vi "Test Pick and Place.vi"() -> ()   [LabVIEW 2011]
uses:
  Config Manager Class/Type Definitions/Fiducial Type.ctl
  Config Manager Class/Type Definitions/Part Type.ctl
  Gantry Class/Gantry Class.lvclass
  CameraTool Class/CameraTool Class.lvclass
  WorkTable Class/WorkTable Class.lvclass
  PickerTool Class.lvclass
  Config Manager Class/Config Manager Class.lvclass
panel:
  out "error out":errorcluster
  in  "BBM Slot":i32
  in  "HDI Slot":i32
  in  "BBM Chuck":i32=1
  in  "HDI Chuck":i32=4
  in  "Virtual Mode":bool
  in  "Config Folder":path=path "C:/Users/husker/Desktop/gantry/Config"
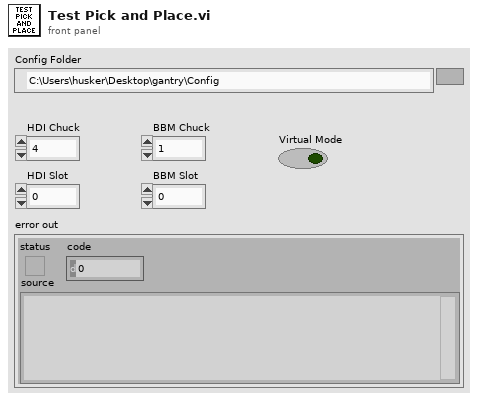
[diagram p1: front panel]
types:
  T1 = typedef "Fiducial Type.ctl" = enum16{"HDI", "BBM"}
  T2 = typedef "Part Type.ctl" = enum16{"BBM", "HDI", "BARE HDI", "GLUERESERVOIR", "STAMP_1", "STAMP_2", "STAMP_3", "STAMP_4", "STAMP_5", "WEIGHT_1", "WEIGHT_2", "WEIGHT_3", "WEIGHT_4", "WEIGHT_5", "WEIGHT_6", "WEIGHT_7", "WEIGHT_8", "PICKER_TOOL", "GRABER_TOOL"}
  T3 = enum16{"Empty", "Bare HDI", "Unglued", "Stamped", "PartOnTop", "Weighted", "Unpotted", "Potted"}
  T4 = cluster{"Feature Coordinates":refnum<class "Vec3d Class.lvclass">, "Feature Name":string}[]
  T5 = typedef "Fiducial Image.ctl" = cluster{"Fiducial Image":T6, "Selected Fiducial":T8, "fiducial name":string}
  T6 = typedef "Physical Image.ctl" = cluster{"Image Position":refnum<class "Vec3d Class.lvclass">, "Image Reference":T7, "Field of View":cluster{"x(mm)":dbl, "y(mm)":dbl}}
  T7 = typedef "IMAQ Image.ctl" = refnum<image>
  T8 = typedef "Fiducial with Source.ctl" = cluster{"Fiducial Image Coordinate":refnum<class "Vec3d Class.lvclass">, "Fiducial Source":enum16{"Pattern Recognition", "User", "Error", "Default"}}
  T9 = typedef "Position_Orientation.ctl" = cluster{"Center":refnum<class "Vec3d Class.lvclass">, "Orientation":refnum<class "Orient3d Class.lvclass">}
  T10 = typedef "Worktable_Module Slot.ctl" = cluster{"Slot State":enum16{"Empty", "Bare HDI", "Unglued", "Stamped", "PartOnTop", "Weighted", "Unpotted", "Potted"}, "BBM Type":enum16{"None", "BBM", "GlassSlide"}, "HDI Type":enum16{"None", "HDI", "Polyimide"}, "Vacuum Channel":u8, "Location/Orientation BBM":T9, "Location/Orientation HDI":T9, "S/N":string}
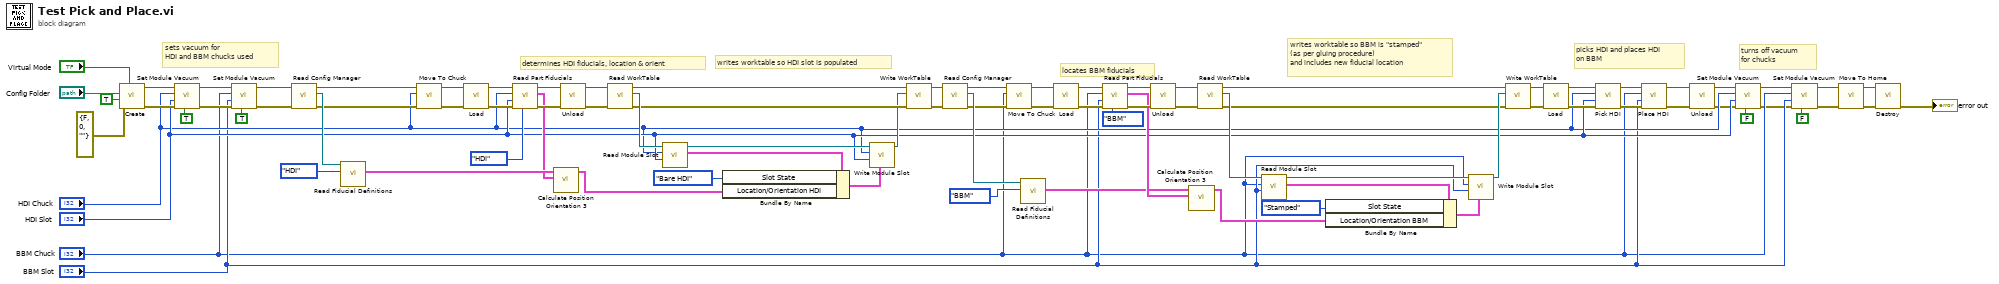
[diagram p0: block diagram]
diagram:
  # "turns off vacuum\nfor chucks"
  # "picks HDI and places HDI\non BBM"
  # "locates BBM fiducials"
  # "determines HDI fiducials, location & orient"
  # "writes worktable so BBM is \"stamped\"\n(as per gluing procedure)\nand includes new fiducial location"
  # "writes worktable so HDI slot is populated"
  # "sets vacuum for \nHDI and BBM chucks used"
  n1 = call "Create.vi"("Virtual Mode"="Virtual Mode", "error in"=errorcluster {"status"=FALSE, "code"=0, "source"=""}, "HOME?"=TRUE, "Config Folder"="Config Folder") -> ("error out"=w80:errorcluster, "Gantry out"=w82:refnum<class "Gantry Class.lvclass">)  [unwired: 6 in]
  n2 = call-dynamic "Set Module Vacuum.vi"("On/Off"=TRUE, "error in"=w80, "Slot Number"="HDI Slot", "Chuck Number"="HDI Chuck", "Gantry in"=w82) -> ("error out"=w79:errorcluster, "Gantry out"=w81:refnum<class "Gantry Class.lvclass">)  [unwired: 5 in]
  n3 = call-dynamic "Set Module Vacuum.vi"("On/Off"=TRUE, "error in"=w79, "Slot Number"="BBM Slot", "Chuck Number"="BBM Chuck", "Gantry in"=w81) -> ("error out"=w51:errorcluster, "Gantry out"=w52:refnum<class "Gantry Class.lvclass">)  [unwired: 5 in]
  n4 = call-dynamic "Read Config Manager.vi"("error in"=w51, "Gantry in"=w52) -> ("error out"=w73:errorcluster, "Config Manager"=w76:refnum<class "Config Manager Class.lvclass">, "Gantry out"=w74:refnum<class "Gantry Class.lvclass">)  [unwired: 7 in]
  n5 = call "Read Fiducial Definitions.vi"("Fiducial Type"=Fiducial_Type."HDI", "Config Manager in"=w76) -> ("Feature Definitions"=w65:T4)  [unwired: 7 in, 2 out]
  n6 = call-dynamic "Move To Chuck.vi"("error in"=w73, "Chuck"="HDI Chuck", "Gantry in"=w74) -> ("error out"=w71:errorcluster, "Gantry out"=w72:refnum<class "Gantry Class.lvclass">)  [unwired: 7 in]
  n7 = call "Load.vi"("error in"=w71, "Gantry In"=w72) -> ("error out"=w69:errorcluster, "CameraTool out"=w70:refnum<class "CameraTool Class.lvclass">)  [unwired: 8 in]
  n8 = call-dynamic "Read Part Fiducials.vi"("Part Type"=Part_Type."HDI", "error in"=w69, "Slot"="HDI Slot", "Chuck"="HDI Chuck", "CameraTool in"=w70) -> ("error out"=w66:errorcluster, "Fiducials"=w64:T5[], "CameraTool out"=w67:refnum<class "CameraTool Class.lvclass">)  [unwired: 4 in]
  n9 = call "Calculate Position Orientation 3.vi"("Fiducials"=w64, "Feature Definitions"=w65) -> ("PositionOrientation"=w47:T9)  [unwired: 8 in, 1 out]
  n10 = call "Unload.vi"("error in"=w66, "CameraTool in"=w67) -> ("error out"=w49:errorcluster, "Gantry out"=w50:refnum<class "Gantry Class.lvclass">)  [unwired: 8 in]
  n11 = call-dynamic "Read WorkTable.vi"("error in"=w49, "Gantry Class in"=w50) -> ("error out"=w53:errorcluster, "WorkTable Class.lvclass"=w56:refnum<class "WorkTable Class.lvclass">, "Gantry Class out"=w54:refnum<class "Gantry Class.lvclass">)  [unwired: 7 in]
  n12 = call-dynamic "Read Module Slot.vi"("slot"="HDI Slot", "chuck"="HDI Chuck", "WorkTable in"=w56) -> ("Module Slot"=w63:T10, "WorkTable out"=w60:refnum<class "WorkTable Class.lvclass">)  [unwired: 6 in, 1 out]
  n13 = Bundle By Name(cluster=w63, "Slot State"=T3."Bare HDI", "Location/Orientation HDI"=w47) -> (w61:T10)
  n14 = call-dynamic "Write Module Slot.vi"("Module Slot"=w61, "slot"="HDI Slot", "chuck"="HDI Chuck", "WorkTable in"=w60) -> ("WorkTable out"=w48:refnum<class "WorkTable Class.lvclass">)  [unwired: 6 in, 1 out]
  n15 = call-dynamic "Write WorkTable.vi"("error in (no error)"=w53, "WorkTable Class.lvclass"=w48, "Gantry Class in"=w54) -> ("error out"=w33:errorcluster, "Gantry Class out"=w37:refnum<class "Gantry Class.lvclass">)  [unwired: 7 in]
  n16 = call-dynamic "Read Config Manager.vi"("error in"=w33, "Gantry in"=w37) -> ("error out"=w32:errorcluster, "Config Manager"=w35:refnum<class "Config Manager Class.lvclass">, "Gantry out"=w36:refnum<class "Gantry Class.lvclass">)  [unwired: 7 in]
  n17 = call-dynamic "Move To Chuck.vi"("error in"=w32, "Chuck"="BBM Chuck", "Gantry in"=w36) -> ("error out"=w45:errorcluster, "Gantry out"=w46:refnum<class "Gantry Class.lvclass">)  [unwired: 7 in]
  n18 = call "Read Fiducial Definitions.vi"("Fiducial Type"=Fiducial_Type."BBM", "Config Manager in"=w35) -> ("Feature Definitions"=w31:T4)  [unwired: 7 in, 2 out]
  n19 = call "Load.vi"("error in"=w45, "Gantry In"=w46) -> ("error out"=w26:errorcluster, "CameraTool out"=w44:refnum<class "CameraTool Class.lvclass">)  [unwired: 8 in]
  n20 = call-dynamic "Read Part Fiducials.vi"("Part Type"=Part_Type."BBM", "error in"=w26, "Slot"="BBM Slot", "Chuck"="BBM Chuck", "CameraTool in"=w44) -> ("error out"=w42:errorcluster, "Fiducials"=w38:T5[], "CameraTool out"=w43:refnum<class "CameraTool Class.lvclass">)  [unwired: 4 in]
  n21 = call "Unload.vi"("error in"=w42, "CameraTool in"=w43) -> ("error out"=w39:errorcluster, "Gantry out"=w40:refnum<class "Gantry Class.lvclass">)  [unwired: 8 in]
  n22 = call "Calculate Position Orientation 3.vi"("Fiducials"=w38, "Feature Definitions"=w31) -> ("PositionOrientation"=w28:T9)  [unwired: 8 in, 1 out]
  n23 = call-dynamic "Read WorkTable.vi"("error in"=w39, "Gantry Class in"=w40) -> ("error out"=w25:errorcluster, "WorkTable Class.lvclass"=w29:refnum<class "WorkTable Class.lvclass">, "Gantry Class out"=w30:refnum<class "Gantry Class.lvclass">)  [unwired: 7 in]
  n24 = call-dynamic "Read Module Slot.vi"("slot"="BBM Slot", "chuck"="BBM Chuck", "WorkTable in"=w29) -> ("Module Slot"=w57:T10, "WorkTable out"=w55:refnum<class "WorkTable Class.lvclass">)  [unwired: 6 in, 1 out]
  n25 = Bundle By Name(cluster=w57, "Slot State"=T3."Stamped", "Location/Orientation BBM"=w28) -> (w59:T10)
  n26 = call-dynamic "Write Module Slot.vi"("Module Slot"=w59, "slot"="BBM Slot", "chuck"="BBM Chuck", "WorkTable in"=w55) -> ("WorkTable out"=w27:refnum<class "WorkTable Class.lvclass">)  [unwired: 6 in, 1 out]
  n27 = call-dynamic "Write WorkTable.vi"("error in (no error)"=w25, "WorkTable Class.lvclass"=w27, "Gantry Class in"=w30) -> ("error out"=w23:errorcluster, "Gantry Class out"=w24:refnum<class "Gantry Class.lvclass">)  [unwired: 7 in]
  n28 = call "Load.vi"("error in"=w23, "Gantry in"=w24) -> ("error out"=w21:errorcluster, "PickerTool out"=w22:refnum<class "PickerTool Class.lvclass">)  [unwired: 8 in]
  n29 = call-dynamic "Pick HDI.vi"("error in"=w21, "Slot"="HDI Slot", "Chuck"="HDI Chuck", "PickerTool in"=w22) -> ("error out"=w19:errorcluster, "PickerTool out"=w20:refnum<class "PickerTool Class.lvclass">)  [unwired: 6 in]
  n30 = call-dynamic "Place HDI.vi"("error in"=w19, "Slot Number"="BBM Slot", "Chuck Number"="BBM Chuck", "PickupTool in"=w20) -> ("error out"=w17:errorcluster, "PickupTool out"=w18:refnum<class "PickerTool Class.lvclass">)  [unwired: 6 in]
  n31 = call "Unload.vi"("error in"=w17, "PickupTool in"=w18) -> ("error out"=w9:errorcluster, "Gantry out"=w10:refnum<class "Gantry Class.lvclass">)  [unwired: 8 in]
  n32 = call-dynamic "Set Module Vacuum.vi"("On/Off"=FALSE, "error in"=w9, "Slot Number"="HDI Slot", "Chuck Number"="HDI Chuck", "Gantry in"=w10) -> ("error out"=w7:errorcluster, "Gantry out"=w8:refnum<class "Gantry Class.lvclass">)  [unwired: 5 in]
  n33 = call-dynamic "Set Module Vacuum.vi"("On/Off"=FALSE, "error in"=w7, "Slot Number"="BBM Slot", "Chuck Number"="BBM Chuck", "Gantry in"=w8) -> ("error out"=w5:errorcluster, "Gantry out"=w6:refnum<class "Gantry Class.lvclass">)  [unwired: 5 in]
  n34 = call-dynamic "Move To Home.vi"("error in"=w5, "Gantry in"=w6) -> ("error out"=w3:errorcluster, "Gantry out"=w4:refnum<class "Gantry Class.lvclass">)  [unwired: 8 in]
  n35 = call "Destroy.vi"("error in"=w3, "Gantry Class in"=w4) -> ("error out"=→"error out":errorcluster)  [unwired: 9 in]
